vi "Install as Service.vi"() -> ()   [LabVIEW 2011]
doc: "Installs an application .exe as a service.\n\n\nVersion 1.0 - 02/13/2013\n\nPhaeron, Inc.\nwww.phaeron.com\ninfo@phaeron.com"
panel:
  in  "SrvAny.exe Path":path=path "c:/Program Files/Windows Resource Kits/Tools/srvany.exe"
  in  "Application Path":path
  in  "Service Name":string
  # "See http://support.microsoft.com/kb/137890"
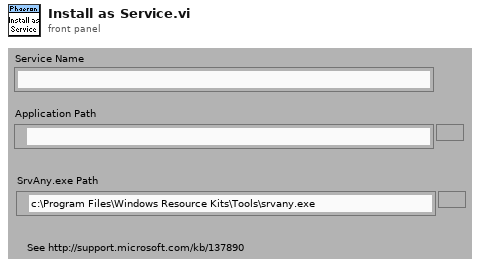
[diagram p1: front panel]
types:
  T1 = enum16{"open", "replace", "create", "open or create", "replace or create", "replace or create with confirmation"}
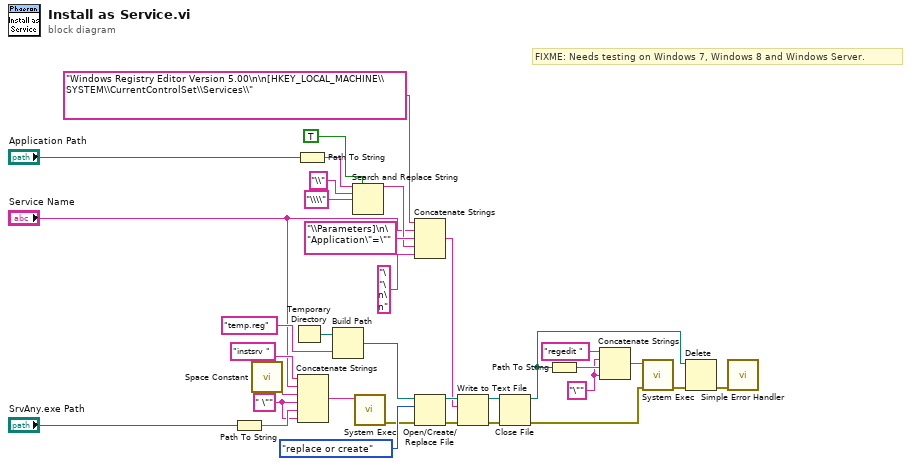
[diagram p0: block diagram]
diagram:
  w2 = " \"" ("string")
  w1 = "\"" ("string")
  # "FIXME: Needs testing on Windows 7, Windows 8 and Windows Server."
  n1 = Path To String(path="SrvAny.exe Path") -> (string=w3:string)
  n2 = call <vilib>:"Space Constant.vi"() -> ("String"=w14:string)
  n3 = Temporary Directory() -> (w34:path)
  n4 = Path To String(path="Application Path") -> (string=w22:string)
  n5 = Concatenate Strings("instsrv " ("string"), "Service Name", w14, w2, w3, w2) -> (w17:string)
  n6 = Build Path(base path=w34, name or relative path="temp.reg") -> (appended path=w5:path)
  n7 = Search and Replace String(replace all?=TRUE ("replace all? (F)"), input string=w22, search string="\\", replace string="\\\\" ("replace string (\"\")")) -> (result string=w18:string)  [unwired: 1 in, 6 out]
  n8 = call <vilib>:"System Exec.vi"("command line"=w17) -> ("error out"=w12:errorcluster)  [unwired: 5 in, 5 out]
  n9 = Concatenate Strings("Windows Registry Editor Version 5.00\n\n[HKEY_LOCAL_MACHINE\\SYSTEM\\CurrentControlSet\\Services\\" ("text"), "Service Name", "\\Parameters]\n\"Application\"=\"" ("text"), w18, "\"\n\n" ("text")) -> (w25:string)
  n10 = Open/Create/Replace File(file path (use dialog)=w5, error in=w12, operation (0:open)=T1."replace or create") -> (refnum out=w30:refnum<file>, error out=w31:errorcluster)  [unwired: 3 in, 1 out]
  n11 = Write to Text File(file (use dialog)=w30, text=w25, error in=w31) -> (refnum out=w23:refnum<file>, error out=w24:errorcluster)  [unwired: 2 out]
  n12 = Close File(refnum=w23, error in=w24) -> (path=w4:path, error out=w11:errorcluster)
  n13 = Path To String(path=w4) -> (string=w8:string)
  n14 = Concatenate Strings("regedit " ("string"), w1, w8, w1) -> (w6:string)
  n15 = call <vilib>:"System Exec.vi"("error in (no error)"=w11, "command line"=w6) -> ("error out"=w10:errorcluster)  [unwired: 4 in, 5 out]
  n16 = Delete(path (use dialog)=w4, error in=w10) -> (error out=w9:errorcluster)  [unwired: 5 out]
  n17 = call <vilib>:"Simple Error Handler.vi"("error in (no error)"=w9) -> ()  [unwired: 1 in, 8 out]
